vi "标定授权发送.vi"(0 "CAN卡类型":u16(ring)=4 items=["PCI5121"=1, "PCI9810"=2, "USBCAN1"=3, "USBCAN2"=4, "PCI9820"=5, "CAN232"=6, "PCI5110"=7, "CANLite(mini)"=8, "ISA9620"=9, "ISA5420"=10, "PC104CAN"=11, "CANETE"=12, "DNP9810"=13], 1 "解锁类型":enum16{"读取", "写", "下载"}(ring), 5 "设备索引号":u16(ring) items=["0", "1", "2", "3", "4", "5", "6", "7", "8", "9", "10", "11", "12", "13", "14", "15", ""], 7 "CAN端口":u16(ring) items=["0", "1"], 9 "是否连接":bool, 11 "板选择":i32 format="%x", 12 "FUNC":u32 format="%x") -> (15 "发送成功":bool=TRUE)   [LabVIEW 2013]
uses:
  data/ControlCAN.dll
panel:
  out "返回类型":u32
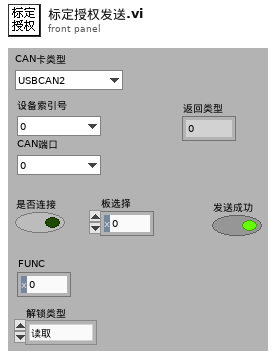
[diagram p1: front panel]
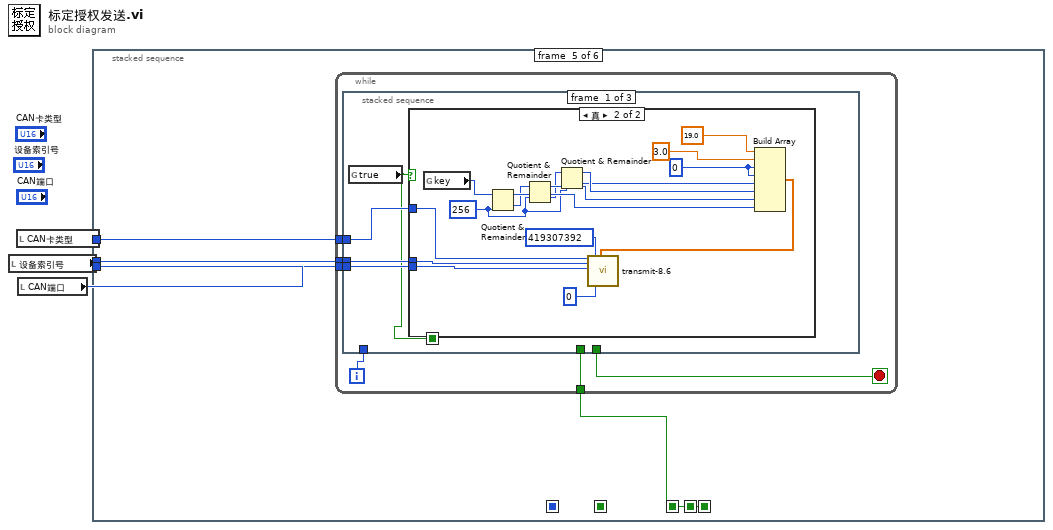
[diagram p0: block diagram]
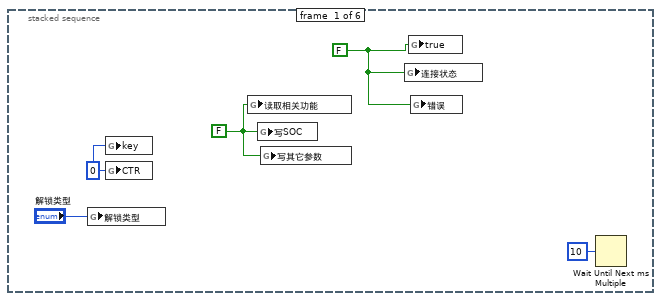
[diagram p2: hidden frame]
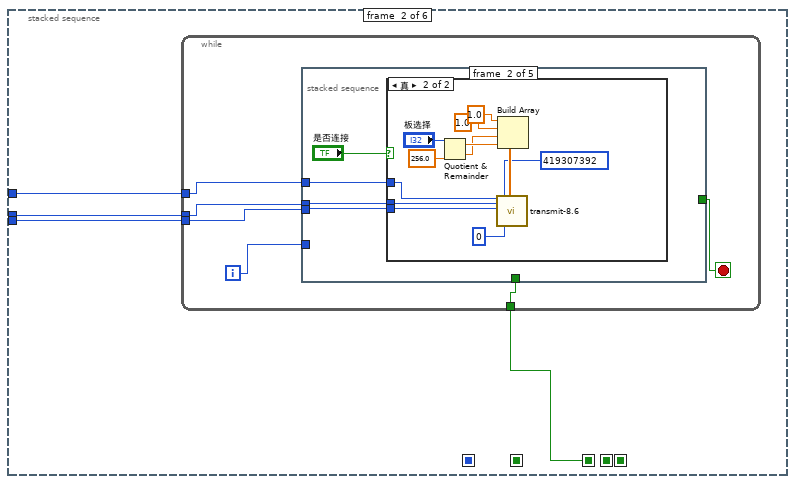
[diagram p3: hidden frame]
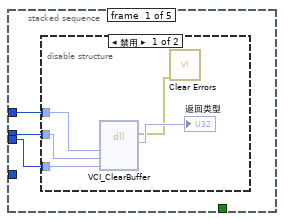
[diagram p4: hidden frame]
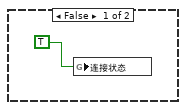
[diagram p6: hidden frame]
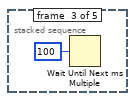
[diagram p7: hidden frame]
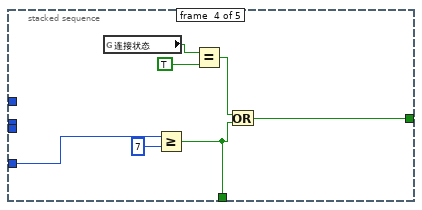
[diagram p8: hidden frame]
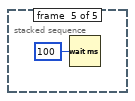
[diagram p9: hidden frame]
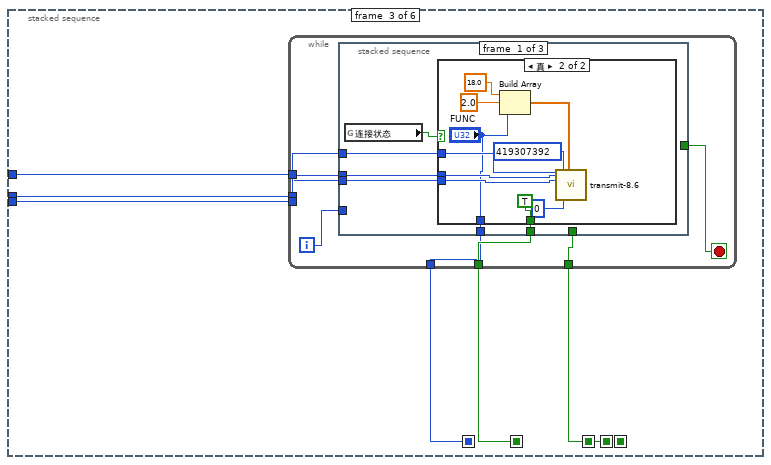
[diagram p10: hidden frame]
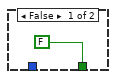
[diagram p11: hidden frame]
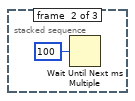
[diagram p12: hidden frame]
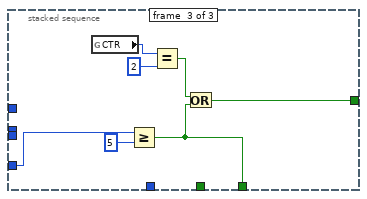
[diagram p13: hidden frame]
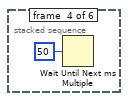
[diagram p14: hidden frame]
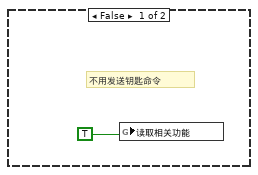
[diagram p15: hidden frame]
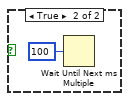
[diagram p17: hidden frame]
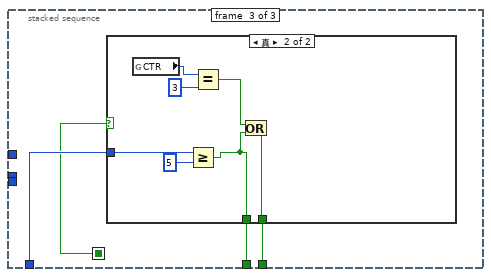
[diagram p18: hidden frame]
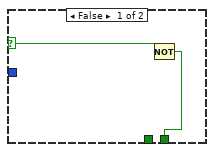
[diagram p19: hidden frame]
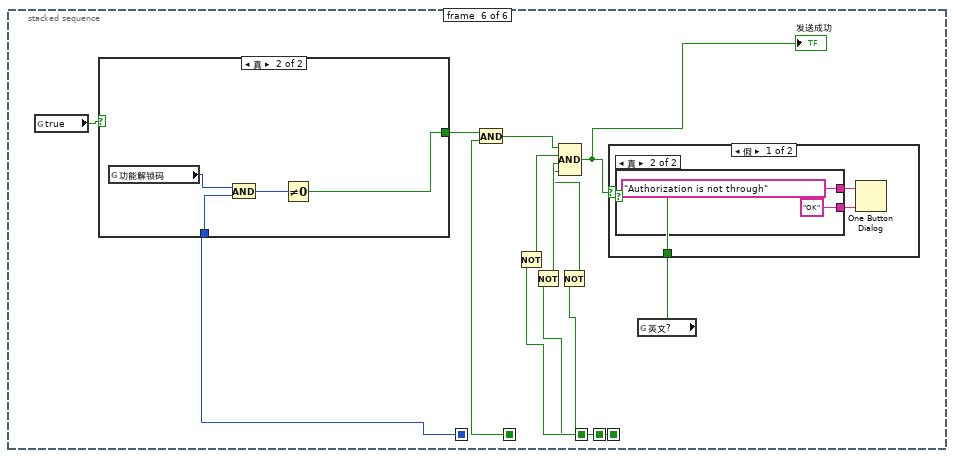
[diagram p20: hidden frame]
diagram:
  n1 = local read "设备索引号"() -> (w2:u16)
  n2 = local read "CAN卡类型"() -> (w3:u16)
  n3 = local read "CAN端口"() -> (w1:u16)
  n4 = stacked-sequence {
    seq-local: [_ _ w55 _ _ _] -> [_ _ _ _ _ w152]
    seq-local: [_ _ w54 _ _ _] -> [_ _ _ _ _ w151]
    seq-local: [_ w9 _ _ _ _] -> [_ _ _ _ _ w150]
    seq-local: [_ _ w53 _ _ _] -> [_ _ _ _ _ w149]
    seq-local: [_ _ _ _ w93 _] -> [_ _ _ _ _ w148]
    tunnel: w3 -> [_ w12 w58 _ w96 _]
    tunnel: w2 -> [_ w11 w57 _ w95 _]
    tunnel: w1 -> [_ w10 w56 _ w94 _]
    frame #0 {
      w6 = FALSE ("连接状态")
      w5 = FALSE ("读取相关功能")
      w7 = u8 0 ("CTR")
      n5 = global write "标定授权全局.vi" "解锁类型"("解锁类型") -> ()
      n6 = global write "标定授权全局.vi" "key"(w7) -> ()
      n7 = global write "标定授权全局.vi" "CTR"(w7) -> ()
      n8 = global write "标定授权全局.vi" "读取相关功能"(w6) -> ()
      n9 = global write "标定授权全局.vi" "写SOC"(w6) -> ()
      n10 = global write "标定授权全局.vi" "写其它参数"(w6) -> ()
      n11 = global write "标定授权全局.vi" "连接状态"(w5) -> ()
      n12 = global write "标定授权全局.vi" "true"(w5) -> ()
      n13 = global write "标定授权全局.vi" "错误"(w5) -> ()
      n14 = Wait Until Next ms Multiple(millisecond multiple=u32 10 ("毫秒倍数")) -> ()  [unwired: 1 out]
    }
    frame #1 {
      n15 = while {
        tunnel: w12 -> [w18]
        tunnel: w11 -> [w17]
        tunnel: w10 -> [w16]
        tunnel: [w13] -> w9
        i -> [w15]
        stop <- w14 stop-if-true
        n16 = stacked-sequence {
          tunnel: w18 -> [w21 w30 _ _ _]
          tunnel: w17 -> [w20 w29 _ _ _]
          tunnel: w16 -> [w19 w28 _ _ _]
          tunnel: w15 -> [_ _ _ w49 _]
          tunnel: [_ _ _ w46 _] -> w14
          tunnel: [_ _ _ w45 _] -> w13
          frame #0 {
            n17 = disable-structure shown="禁用" {
              disable-tunnel: w21 -> [w26 _]
              disable-tunnel: w20 -> [w25 _]
              disable-tunnel: w19 -> [w24 _]
              frame Disabled {
                n18 = dll-call lib="PTH1Eabs EEV05EV05监控上位机-EV05EV05dataControlCAN.dll" fn="VCI_ClearBuffer"("DeviceType"=w26, "DeviceInd"=w25, "CANInd"=w24) -> (error out=w22:errorcluster, "返回类型"=→"返回类型":u32)  [unwired: 4 in, 3 out]
                n19 = call <vilib>:"Clear Errors.vi"("error in (no error)"=w22) -> ()  [unwired: 6 in, 1 out]
              }
              frame Enabled {
              }
            }
          }
          frame #1 {
            n20 = case shown="真" "是否连接" {
              tunnel: w30 -> [_ w35]
              tunnel: w29 -> [_ w34]
              tunnel: w28 -> [_ w33]
              frame False {
                n21 = global write "标定授权全局.vi" "连接状态"(TRUE ("连接状态")) -> ()
              }
              frame True {
                n22 = Quotient & Remainder(x="板选择", y=256.0) -> (x-y*floor(x/y)=w43:dbl, floor(x/y)=w42:dbl)
                n23 = Build Array(1.0 ("元素"), 1.0 ("元素"), w42, w43) -> (w38:dbl[])
                n24 = call "transmit-8.6.vi"("can卡类型"=w35, "设备索引号"=w34, "CAN端口"=w33, "ID"=u32 419307392, "SendType"=u8 0, "Data"=w38) -> ()  [unwired: 3 in, 11 out]
              }
            }
          }
          frame #2 {
            n25 = Wait Until Next ms Multiple(millisecond multiple=u32 100 ("等待时间（毫秒）")) -> ()  [unwired: 1 out]
          }
          frame #3 {
            n26 = global read "标定授权全局.vi" "连接状态"() -> (w51:bool)
            n27 = Greater Or Equal?(x=w49, y=7) -> (x >= y?=w45:bool)
            n28 = Equal?(x=w51, y=TRUE) -> (x = y?=w47:bool)
            n29 = Or(x=w47, y=w45) -> (x .or. y?=w46:bool)
          }
          frame #4 {
            n30 = Wait (ms)(milliseconds to wait=u32 100 ("等待时间（毫秒）")) -> ()  [unwired: 1 out]
          }
        }
      }
    }
    frame #2 {
      n31 = while {
        tunnel: w58 -> [w66]
        tunnel: w57 -> [w65]
        tunnel: w56 -> [w64]
        tunnel: [w63] -> w55
        tunnel: [w62] -> w54
        tunnel: [w59] -> w53
        i -> [w61]
        stop <- w60 stop-if-true
        n32 = stacked-sequence {
          tunnel: w66 -> [w72 _ _]
          tunnel: w65 -> [w71 _ _]
          tunnel: w64 -> [w70 _ _]
          tunnel: [w68 _ _] -> w63
          tunnel: [w67 _ _] -> w62
          tunnel: w61 -> [_ _ w89]
          tunnel: [_ _ w87] -> w60
          tunnel: [_ _ w86] -> w59
          frame #0 {
            n33 = global read "标定授权全局.vi" "连接状态"() -> (w69:bool)
            n34 = case shown="真" w69 {
              tunnel: w72 -> [_ w77]
              tunnel: w71 -> [_ w83]
              tunnel: w70 -> [_ w82]
              tunnel: [FALSE TRUE] -> w68
              tunnel: [_ "FUNC"] -> w67
              frame False {
              }
              frame True {
                n35 = Build Array(18.0 ("元素"), 2.0 ("元素"), "FUNC") -> (w78:dbl[])
                n36 = call "transmit-8.6.vi"("can卡类型"=w77, "设备索引号"=w83, "CAN端口"=w82, "ID"=u32 419307392, "SendType"=u8 0, "Data"=w78) -> ()  [unwired: 3 in, 11 out]
              }
            }
          }
          frame #1 {
            n37 = Wait Until Next ms Multiple(millisecond multiple=u32 100 ("等待时间（毫秒）")) -> ()  [unwired: 1 out]
          }
          frame #2 {
            n38 = global read "标定授权全局.vi" "CTR"() -> (w91:u8)
            n39 = Greater Or Equal?(x=w89, y=5) -> (x >= y?=w86:bool)
            n40 = Equal?(x=w91, y=u8 2) -> (x = y?=w85:bool)
            n41 = Or(x=w85, y=w86) -> (x .or. y?=w87:bool)
          }
        }
      }
    }
    frame #3 {
      n42 = Wait Until Next ms Multiple(millisecond multiple=u32 50 ("毫秒倍数")) -> ()  [unwired: 1 out]
    }
    frame #4 {
      n43 = while {
        tunnel: w96 -> [w102]
        tunnel: w95 -> [w101]
        tunnel: w94 -> [w100]
        tunnel: [w97] -> w93
        i -> [w99]
        stop <- w98 stop-if-true
        n44 = stacked-sequence {
          seq-local: [w103 _ _] -> [_ w125 w128]
          tunnel: w102 -> [w106 _ _]
          tunnel: w101 -> [w105 _ _]
          tunnel: w100 -> [w104 _ _]
          tunnel: w99 -> [_ _ w130]
          tunnel: [_ _ w129] -> w98
          tunnel: [_ _ w127] -> w97
          frame #0 {
            n45 = global read "标定授权全局.vi" "true"() -> (w103:bool)
            n46 = case shown="真" w103 {
              tunnel: w106 -> [_ w124]
              tunnel: w105 -> [_ w123]
              tunnel: w104 -> [_ w122]
              frame False {
                # "不用发送钥匙命令"
                n47 = global write "标定授权全局.vi" "读取相关功能"(TRUE ("读取相关功能")) -> ()
              }
              frame True {
                w109 = 0
                w112 = u32 256 ("y")
                n48 = global read "标定授权全局.vi" "key"() -> (w111:u32)
                n49 = Quotient & Remainder(x=w111, y=w112) -> (x-y*floor(x/y)=w117:u32, floor(x/y)=w116:u32)
                n50 = Quotient & Remainder(x=w116, y=w112) -> (x-y*floor(x/y)=w115:u32, floor(x/y)=w114:u32)
                n51 = Quotient & Remainder(x=w114, y=w112) -> (x-y*floor(x/y)=w113:u32, floor(x/y)=w110:u32)
                n52 = Build Array(19.0 ("元素"), 3.0 ("元素"), w109, w109, w110, w113, w115, w117) -> (w118:dbl[])
                n53 = call "transmit-8.6.vi"("can卡类型"=w124, "设备索引号"=w123, "CAN端口"=w122, "ID"=u32 419307392, "SendType"=u8 0, "Data"=w118) -> ()  [unwired: 3 in, 11 out]
              }
            }
          }
          frame #1 {
            n54 = case shown="假" w125 {
              frame False {
              }
              frame True {
                n55 = Wait Until Next ms Multiple(millisecond multiple=u32 100 ("等待时间（毫秒）")) -> ()  [unwired: 1 out]
              }
            }
          }
          frame #2 {
            n56 = case shown="真" w128 {
              selector: w128 -> [w131 _]
              tunnel: w130 -> [_ w137]
              tunnel: [w132 w134] -> w129
              tunnel: [_ w133] -> w127
              frame False {
                n57 = Not(x=w131) -> (.not. x?=w132:bool)
              }
              frame True {
                n58 = global read "标定授权全局.vi" "CTR"() -> (w139:u8)
                n59 = Greater Or Equal?(x=w137, y=5) -> (x >= y?=w133:bool)
                n60 = Equal?(x=w139, y=u8 3) -> (x = y?=w135:bool)
                n61 = Or(x=w135, y=w133) -> (x .or. y?=w134:bool)
              }
            }
          }
        }
      }
    }
    frame #5 {
      n62 = global read "标定授权全局.vi" "true"() -> (w141:bool)
      n63 = case shown="真" w141 {
        tunnel: w151 -> [_ w156]
        tunnel: [TRUE ("写其它参数") w154] -> w147
        frame False {
        }
        frame True {
          n64 = global read "标定授权全局.vi" "功能解锁码"() -> (w157:u8)
          n65 = And(x=w157, y=w156) -> (x .and. y?=w155:u32)
          n66 = Not Equal To 0?(x=w155) -> (x != 0?=w154:bool)
        }
      }
      n67 = And(x=w147, y=w152) -> (x .and. y?=w145:bool)
      n68 = Not(x=w150) -> (.not. x?=w144:bool)
      n69 = Not(x=w149) -> (.not. x?=w143:bool)
      n70 = Not(x=w148) -> (.not. x?=w142:bool)
      n71 = Compound Arithmetic op=AND(w145, w144, w143, w142) -> (w146:bool)
      "发送成功" <- w146
      n72 = global read "中英文全局-8.6.vi" "英文?"() -> (w140:bool)
      n73 = case shown="假" w146 {
        tunnel: w140 -> [w158 _]
        frame False {
          n74 = case shown="真" w158 {
            tunnel: ["授权不通过" ("消息") "Authorization is not through" ("消息")] -> w160
            tunnel: ["是" ("按钮名称（“确定”）") "OK" ("按钮名称（“确定”）")] -> w159
            frame False {
            }
            frame True {
            }
          }
          n75 = One Button Dialog(message=w160, button name ("OK")=w159) -> ()  [unwired: 1 out]
        }
        frame True {
        }
      }
    }
  }
